vi "FT_Write_String_Data.vi"(2 "Buffer":string, 3 "Handle":u32) -> (0 "Bytes Written":u32, 1 "FT_Status":u32)   [LabVIEW 2018]
uses:
  FTD2XX.dll
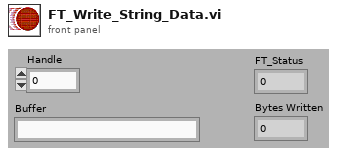
[diagram p1: front panel]
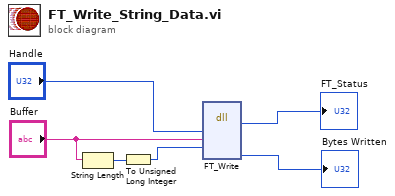
[diagram p0: block diagram]
diagram:
  n1 = String Length(string="Buffer") -> (length=w2:i32)
  n2 = To Unsigned Long Integer(number=w2) -> (unsigned 32bit integer=w1:u32)
  n3 = dll-call lib="FTD2XX.dll" fn="FT_Write"("Handle"="Handle", "Buffer"="Buffer", "BytesToWrite"=w1) -> ("FT_Status"=→"FT_Status":u32, "BytesWritten"=→"Bytes Written":u32)  [unwired: 7 in, 2 out]
